vi "Read TCPIP address.vi"(8 "error in (no error)":errorcluster, 11 "ESP301_via_TCPIP in":refnum<class "ESP301_via_TCPIP.lvclass">) -> (0 "error out":errorcluster, 2 "TCPIP address":refnum<k5>, 3 "ESP301_via_TCPIP out":refnum<class "ESP301_via_TCPIP.lvclass">)   [LabVIEW 2018, in "ESP301_via_TCPIP.lvclass"]
uses:
  ESP301_via_TCPIP.lvclass
  ESP301_via_TCPIP.lvclass/ESP301_via_TCPIP.ctl
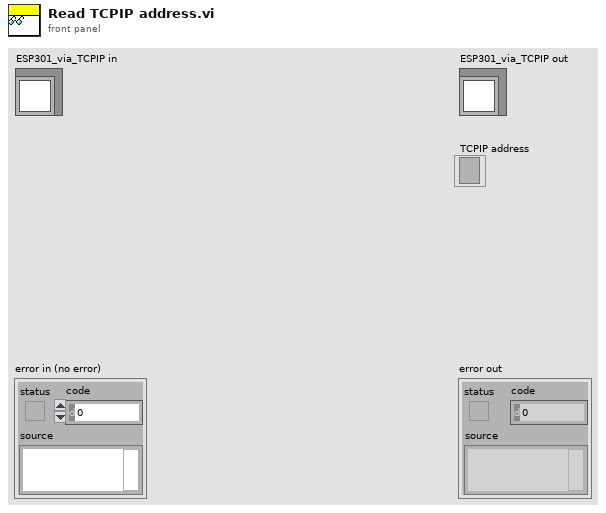
[diagram p1: front panel]
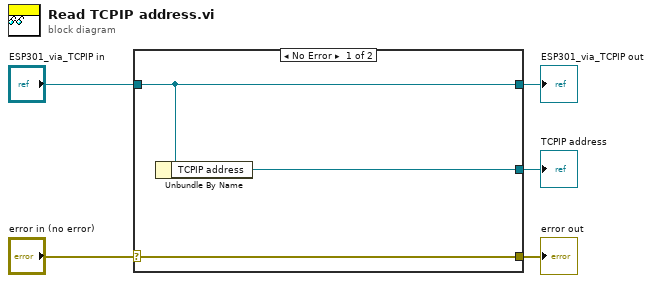
[diagram p0: block diagram]
diagram:
  n1 = case shown="No Error" "error in (no error)" {
    selector: "error in (no error)" -> [w8 w9]
    tunnel: [w8 w9] -> w4
    tunnel: [w7 w10] -> w2
    tunnel: "ESP301_via_TCPIP in" -> [w7 w10]
    tunnel: [w6 _] -> w1
    frame No Error {
      n2 = Unbundle By Name(w7) -> ("TCPIP address"=w6:refnum<k5>)
    }
    frame Error {
    }
  }
  "error out" <- w4
  "ESP301_via_TCPIP out" <- w2
  "TCPIP address" <- w1
